vi "SpecAnReadorFetch.vi"(7 "Set Read/Write (F)":bool, 11 "FetchorRead":bool) -> (3 "Boolean":bool)   [LabVIEW 2018, in "SpecAnModule.lvlib"]
doc: "This VI functions as an action node to pass an enum that determins wether the acquisition is in fetch or read mode."
uses:
  SpecAnModule.lvlib
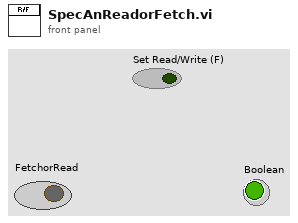
[diagram p1: front panel]
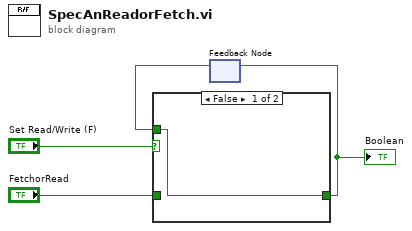
[diagram p0: block diagram]
diagram:
  n1 = feedback #1() -> (w3:bool)  [unwired: 1 in]
  n2 = case shown="False" "Set Read/Write (F)" {
    tunnel: w3 -> [w5 _]
    tunnel: "FetchorRead" -> [_ w6]
    tunnel: [w5 w6] -> w1
    frame False {
    }
    frame True {
    }
  }
  "Boolean" <- w1
  n3 = feedback-in #1(w1) -> ()
